vi "Module Init.vi"(8 "error in (no error)":errorcluster, 11 "HTTP Command Bridge in":refnum<class "HTTP Command Bridge.lvclass">) -> (0 "error out":errorcluster, 3 "HTTP Command Bridge out":refnum<class "HTTP Command Bridge.lvclass">)   [LabVIEW 2020, in "Volatus.lvlib" / "HTTP Command Bridge.lvclass"]
uses:
  HTTP Command Bridge.lvclass
  HTTP Command Bridge.lvclass/HTTP Command Bridge.ctl
  Module/Module.lvclass
  C:/dev/lv20CE/relink/lv-volatus/Volatus/Module/Module.lvclass
  C:/dev/lv20CE/relink/lv-volatus/Volatus/HTTP Command Bridge/HTTP Command Bridge.lvclass
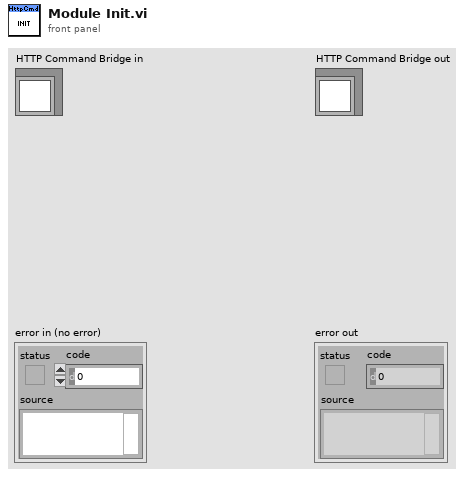
[diagram p1: front panel]
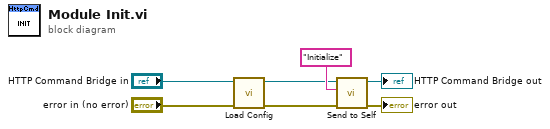
[diagram p0: block diagram]
diagram:
  n1 = call "Load Config.vi"("error in (no error)"="error in (no error)", "HTTP Command Bridge in"="HTTP Command Bridge in") -> ("error out"=w3:errorcluster, "HTTP Command Bridge out"=w1:refnum<class "HTTP Command Bridge.lvclass">)  [unwired: 8 in]
  n2 = call "Send to Self.vi"("error in (no error)"=w3, "Message ID"="Initialize", "Module in"=w1) -> ("error out"=→"error out":errorcluster, "Module in"=→"HTTP Command Bridge out":refnum<class "HTTP Command Bridge.lvclass">)  [unwired: 7 in]
